vi "Pick AI Move.vi"(10 "Team":bool, 11 "AI Table Head":i32) -> (0 "Prob":dbl caption="Selected Probability (Debugging)", 1 "Selected Col":i32, 2 "Selected Row":i32, 3 "AI Table Child":i32)   [LabVIEW 2013]
uses:
  Typedef/AI Table Node.ctl
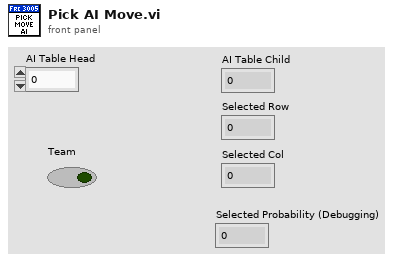
[diagram p1: front panel]
types:
  T1 = typedef "AI Table Node.ctl" = cluster{"Board State":i32, "Child Nodes":i32[], "X PCT":dbl, "O PCT":dbl, "Index":i32}
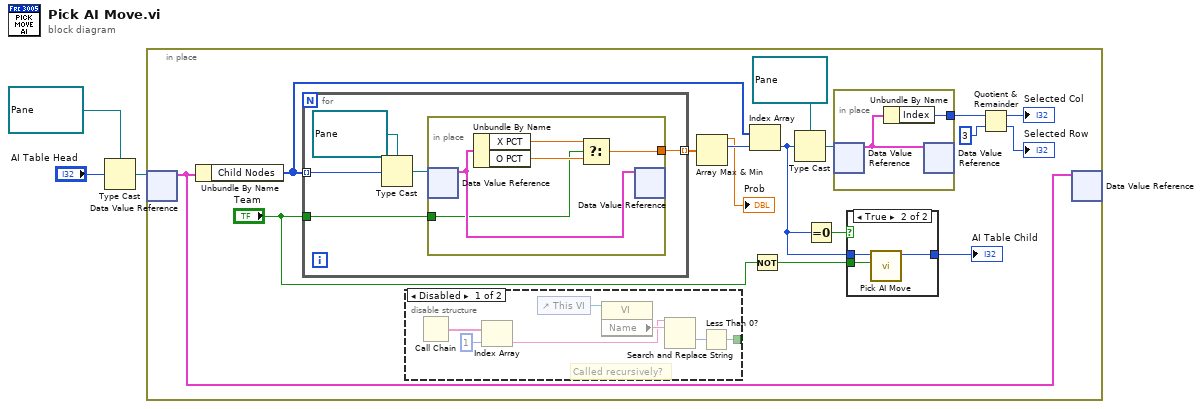
[diagram p0: block diagram]
diagram:
  n1 = Type Cast(type=refnum<data-value> refnum ("data value reference"), x="AI Table Head") -> (*(type *) &x=w3:refnum<data-value>)
  n2 = in-place {
    n3 = in-place-dvr #1(w3) -> (w19:T1)  [unwired: 1 out]
    n4 = Unbundle By Name(w19) -> ("Child Nodes"=w17:i32[])
    n5 = for {
      tunnel: w17 -> [w35] mode=indexing
      tunnel: [w34] -> w18 mode=indexing
      tunnel: "Team" -> [w33]
      n6 = Type Cast(type=refnum<data-value> refnum ("data value reference"), x=w35) -> (*(type *) &x=w36:refnum<data-value>)
      n7 = in-place {
        in-place-border: [w41] -> w34
        in-place-border: w33 -> [w38]
        n8 = in-place-dvr #2(w36) -> (w42:T1)  [unwired: 1 out]
        n9 = Unbundle By Name(w42) -> ("X PCT"=w39:dbl, "O PCT"=w40:dbl)
        n10 = Select(t=w39, s=w38, f=w40) -> (s? t:f=w41:dbl)
        n11 = in-place-dvr #2(w42) -> ()  [unwired: 2 out]
      }
    }
    n12 = disable-structure shown="Disabled" {
      disable-tunnel: [w21 _] -> _
      frame Disabled {
        # "Called recursively?"
        n13 = Call Chain() -> (call chain=w26:string[])
        n14 = Index Array(array=w26, index=1) -> (element=w22:string)
        n15 = control-ref of="This VI"() -> (w23:refnum<vi>)
        n16 = property class="VI"(reference=w23) -> ("Name"=w25:string)  [unwired: 1 in, 2 out]
        n17 = Search and Replace String(input string=w22, search string=w25) -> (offset past replacement=w24:i32)  [unwired: 6 in, 3 out]
        n18 = Less Than 0?(x=w24) -> (x < 0?=w21:bool)
      }
      frame Enabled {
      }
    }
    n19 = Array Max & Min(array=w18) -> (max value=→"Prob":dbl, max index (indices)=w10:i32)  [unwired: 2 out]
    n20 = Index Array(array=w17, index=w10) -> (element=w4:i32)
    n21 = Not(x="Team") -> (.not. x?=w7:bool)
    n22 = Type Cast(type=refnum<data-value> refnum ("data value reference"), x=w4) -> (*(type *) &x=w15:refnum<data-value>)
    n23 = Equal To 0?(x=w4) -> (x = 0?=w5:bool)
    n24 = in-place {
      in-place-border: [w31] -> w14
      n25 = in-place-dvr #3(w15) -> (w32:T1)  [unwired: 1 out]
      n26 = Unbundle By Name(w32) -> ("Index"=w31:i32)
      n27 = in-place-dvr #3(w32) -> ()  [unwired: 2 out]
    }
    n28 = case shown="True" w5 {
      tunnel: w4 -> [w27 w30]
      tunnel: w7 -> [_ w29]
      tunnel: [w27 w28] -> w6
      frame False {
      }
      frame True {
        n29 = call "Pick AI Move.vi"("Team"=w29, "AI Table Head"=w30) -> ("AI Table Child"=w28:i32)  [unwired: 6 in, 3 out]
      }
    }
    "AI Table Child" <- w6
    n30 = Quotient & Remainder(x=w14, y=3) -> (x-y*floor(x/y)=→"Selected Col":i32, floor(x/y)=→"Selected Row":i32)
    n31 = in-place-dvr #1(w19) -> ()  [unwired: 2 out]
  }
